vi "Listen.vi"(8 "error in (no error)":errorcluster, 11 "CIFTemplatePlugin in":refnum<class "TemplatePlugin.lvclass">) -> (0 "error out":errorcluster, 3 "CIFTemplatePlugin out":refnum<class "TemplatePlugin.lvclass">)   [LabVIEW 2021, in "TemplatePlugin.lvclass"]
uses:
  TemplatePlugin.lvclass
  D:/dev/CIF-LVCore/src/CIFCore/Class/CIFCorePlugin.lvclass
  CIF-LVCore/src/CIFCore/Class/Typedef/Energized States.ctl
  CIF-LVCore/src/CIFCore/Class/CIFCorePlugin.lvclass/CIFCorePlugin.ctl
  TemplatePlugin.lvclass/TemplatePlugin.ctl
  <vilib>/CIF Foundation/CIF Utilities/Statistics/I64/Stats_I64_CIF_U.lvclass/Stats_I64_CIF_U.ctl
  CIF-LVCore/src/Channels/CIFChannelMng/CIFChannelMng.lvclass/CIFChannelMng.ctl
  <vilib>/CIF Foundation/CIF Channels Core/CIFChannels/CIFChannels.lvclass/CIFChannels.ctl
  CIF-LVCore/src/CIFCore/Class/SubVIs/OOB/Update Status from Benchmarks.vi
  CIF-LVCore/src/Channels/CIFChannelMng/Core/Send Channel List Update.vi
  CIF-LVCore/src/CIFCore/Class/SubVIs/OOB/Send Core OOB TX.vi/074d8088-3ad4-4fdc-9542-b009f1b06b72.vi
  CIF-LVCore/src/CIFCore/Class/SubVIs/Refresh Stats.vi
  CIF-LVCore/src/CIFCore/Class/SubVIs/OOB/Receive/Read Clock Map.vi
  CIF-LVCore/src/CIFCore/Class/SubVIs/OOB/Receive/Read Connections.vi
  CIF-LVCore/src/Channels/CIFChannelMng/SubVIs/Connect Channel.vi
  CIF-LVCore/src/CIFCore/Class/SubVIs/OOB/Receive/Read Forces.vi
  CIF-LVCore/src/Channels/CIFChannelMng/SubVIs/Force Channel.vi
  CIF-LVCore/src/Channels/CIFChannelMng/SubVIs/Add FIFO Publisher.vi
  CIF-LVCore/src/CIFCore/Class/SubVIs/OOB/Receive/Read Publisher Instance.vi
  CIF-LVCore/src/Channels/CIFChannelMng/Core/Send Publisher Instance Return.vi
  CIF-LVCore/src/Channels/CIFChannelMng/SubVIs/Remove FIFO Publisher.vi
  CIF-LVCore/src/CIFCore/Class/SubVIs/OOB/Read Core OOB RX.vi/a31a91a9-4107-4750-8e0d-44486e9a3a34.vi
  OOB Comm/Read Comm to Main.vi/525c214c-2a6b-4e7b-b3ce-0ad96b412d2f.vi
  OOB Comm/Read Comm to Main.vi/4efb0375-f1de-4191-b03f-44d34e6646cb.vi
  OOB Comm/Send Cyclic to gRPC.vi/0c0f428d-7269-422d-ba27-f9d6fa7232ec.vi
  CIF-LVCore/src/CIFCore/Class/Accessors/Read Refresh.vi
  <vilib>/CIF Foundation/CIF Utilities/Statistics/I64/Get Stats.vi
  CIF-LVCore/src/Channels/CIFChannelMng/Core/Send Channel List Update.vi/463ebf4c-8748-40f9-8ad3-9e61c16a01a6.vi
  <vilib>/CIF Foundation/CIF CIPC/SubVIs/Check Error.vi
  <vilib>/CIF Foundation/CIF CIPC/SubVIs/Get Element Write Position.vi
  <vilib>/CIF Foundation/CIF CIPC/SubVIs/Notify Of New Write.vi
  <vilib>/CIF Foundation/CIF CIPC/SubVIs/Get dll Path.vi
  CIF-LVCore/src/Channels/CIFChannelMng/Utilities/Get Channel Index by Name.vi
  <vilib>/CIF Foundation/CIF Channels Core/CIFChannels/Accessors/Read Channel State.vi
  <vilib>/CIF Foundation/CIF Channels Core/CIFChannels/Accessors/Read Tag Forced.vi
  CIF-LVCore/src/Channels/CIFChannelMng/SubVIs/Add Error Channel Manager.vi
  CIF-LVCore/src/Channels/CIFChannelMng/Core/Send Publisher Instance Return.vi/9db40550-ae0b-4108-a32d-02e81b824dbe.vi
  CIF-LVCore/src/Channels/CIFChannelMng/SubVIs/Get Original FIFO Channel Name.vi
  <vilib>/CIF Foundation/CIF CIPC/SubVIs/Wait For N Elements Available.vi
  <vilib>/CIF Foundation/CIF CIPC/SubVIs/Get Element Read Position.vi
  <vilib>/CIF Foundation/CIF CIPC/SubVIs/Set Element Read Position.vi
  <vilib>/CIF Foundation/CIF Channels Core/ChannelCommon/Utilities/Add Error.vi
  <vilib>/CIF Foundation/CIF Utilities/Errors/Append Error Location.vi
  <vilib>/CIF Foundation/CIF CIPC/SubVIs/Get Element Info Variant.vi
  <vilib>/Utility/error.llb/Trim Whitespace.vi
  <vilib>/Utility/error.llb/Error Cluster From Error Code.vi
  <vilib>/CIF Foundation/CIF Channels Core/CIFChannels/Core/Set Force.vi
  CIF-LVCore/src/CIFCore/Class/CIFCorePlugin.lvclass
  <vilib>/CIF Foundation/CIF Channels Core/CIFChannels/CIFChannels.lvclass
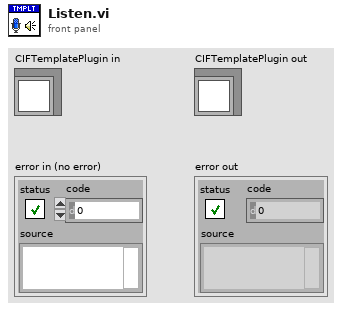
[diagram p1: front panel]
types:
  T1 = typedef "CIFCorePlugin.lvclass/Energized States.ctl" = enum16{"Listen", "Prepare", "Execute", "Housekeep", "Cleanup", "Destroy"}
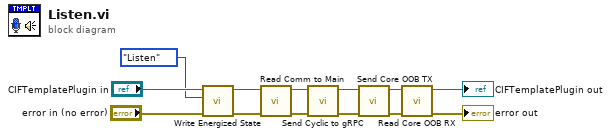
[diagram p0: block diagram]
diagram:
  n1 = call "Write Energized State.vi"("error in (no error)"="error in (no error)", "Energized State"=Energized_States."Listen", "CIFCorePlugin in"="CIFTemplatePlugin in") -> ("error out"=w10:errorcluster, "CIFCorePlugin out"=w11:refnum<class "TemplatePlugin.lvclass">)  [unwired: 7 in]
  n2 = call "Read Comm to Main.vi"("error in (no error)"=w10, "CIFTemplatePlugin in"=w11) -> ("error out"=w2:errorcluster, "CIFTemplatePlugin out"=w1:refnum<class "TemplatePlugin.lvclass">)  [unwired: 8 in]
  n3 = call "Send Cyclic to gRPC.vi"("error in (no error)"=w2, "CIFTemplatePlugin in"=w1) -> ("error out"=w6:errorcluster, "CIFTemplatePlugin out"=w7:refnum<class "TemplatePlugin.lvclass">)  [unwired: 8 in]
  n4 = call "Send Core OOB TX.vi"("error in (no error)"=w6, "CIFCorePlugin in"=w7) -> ("error out"=w8:errorcluster, "CIFCorePlugin out"=w3:refnum<class "TemplatePlugin.lvclass">)  [unwired: 8 in]
  n5 = call "Read Core OOB RX.vi"("error in (no error)"=w8, "CIFCorePlugin in"=w3) -> ("error out"=→"error out":errorcluster, "CIFCorePlugin out"=→"CIFTemplatePlugin out":refnum<class "TemplatePlugin.lvclass">)  [unwired: 8 in]
